vi "List_files_in_order_of_age.vi"(1 "Files to Hide":string[](array[string]), 2 "Folder":path) -> (0 "file names":string[](array[string]))   [LabVIEW 2010]
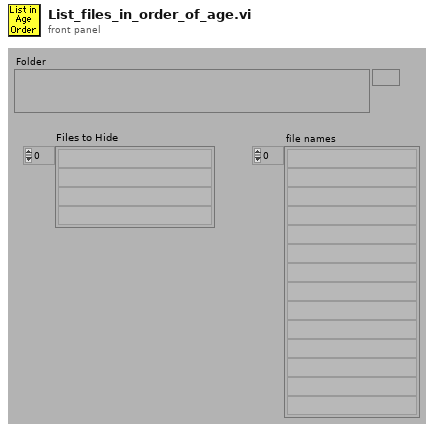
[diagram p1: front panel]
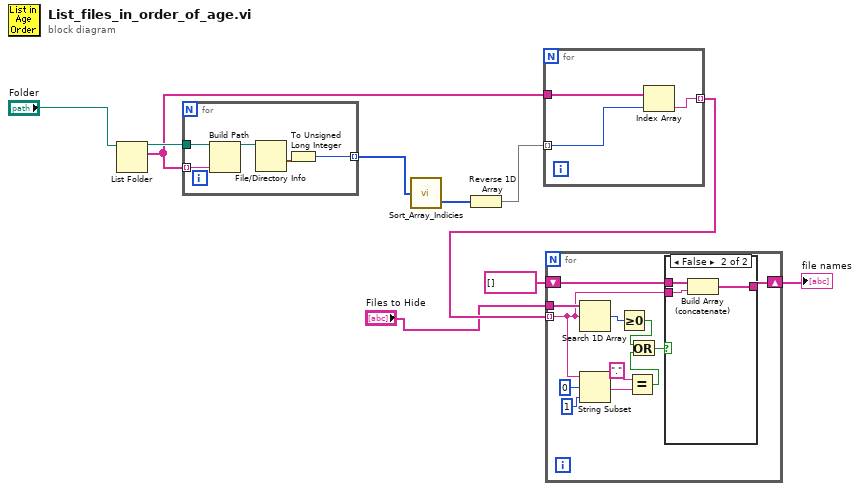
[diagram p0: block diagram]
diagram:
  n1 = List Folder(path="Folder") -> (path out=w9:path, filenames=w8:string[])  [unwired: 1 in, 4 out]
  n2 = for {
    tunnel: w9 -> [w15]
    tunnel: w8 -> [w12] mode=indexing
    tunnel: [w11] -> w1 mode=indexing
    n3 = Build Path(base path=w15, name or relative path=w12) -> (appended path=w14:path)
    n4 = File/Directory Info(path=w14) -> (last mod=w13:timestamp)  [unwired: 1 in, 6 out]
    n5 = To Unsigned Long Integer(number=w13) -> (unsigned 32bit integer=w11:u32)
  }
  n6 = call "Sort_Array_Indicies.vi"("unsorted array"=w1) -> ("Sort Index"=w6:i32[])  [unwired: 1 out]
  n7 = Reverse 1D Array(array=w6) -> (reversed array=w10:i32[])
  n8 = for {
    tunnel: w10 -> [w16] mode=indexing
    tunnel: [w18] -> w5 mode=indexing
    tunnel: w8 -> [w17]
    n9 = Index Array(array=w17, index=w16) -> (element=w18:string)
  }
  n10 = for {
    shift-right: [w28] -> w4
    shift-left: string[] [] -> [w30]
    tunnel: w5 -> [w22] mode=indexing
    tunnel: "Files to Hide" -> [w29]
    n11 = Search 1D Array(1D array=w29, element=w22) -> (index of element=w27:i32)  [unwired: 1 out]
    n12 = String Subset(string=w22, offset (0)=0, length (rest)=1 ("length")) -> (substring=w25:string)
    n13 = Greater Or Equal To 0?(x=w27) -> (x >= 0?=w21:bool)
    n14 = Equal?(x=".", y=w25) -> (x = y?=w20:bool)
    n15 = Or(x=w21, y=w20) -> (x .or. y?=w19:bool)
    n16 = case shown="False" w19 {
      tunnel: w30 -> [w31 w34]
      tunnel: [w31 w33] -> w28
      tunnel: w22 -> [_ w32]
      frame True {
      }
      frame False {
        n17 = Build Array (concatenate)(w34, w32) -> (w33:string[])
      }
    }
  }
  "file names" <- w4
